vi "ForkOpening.vi"(9 "Presets":T2, 10 "Buttons":bool[](array[boolean])) -> (2 "Opening":T1)   [LabVIEW 2014]
doc: "Set the fork opening according to the button position. Set ForkOffset too"
uses:
  buttons/PresetValues.ctl
  ForkOpening.ctl
  <vilib>/Rock Robotics/Network Tables/SD Write Number.vi
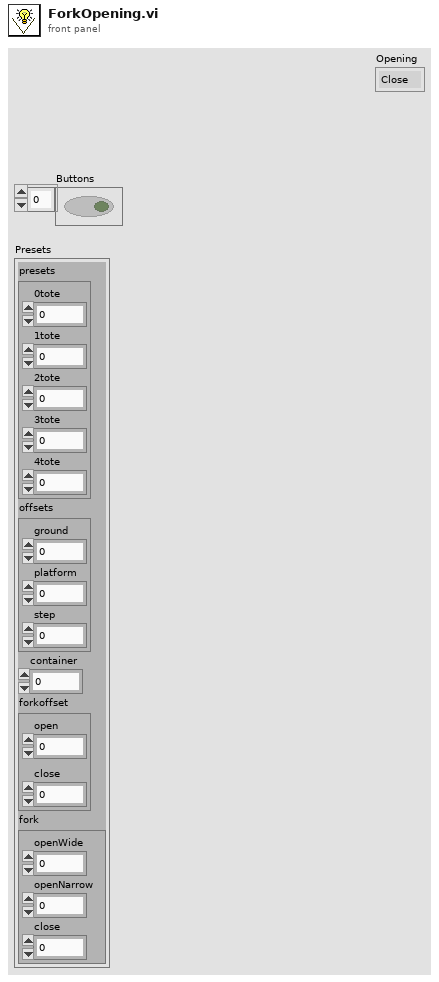
[diagram p1: front panel]
types:
  T1 = typedef "ForkOpening.ctl" = enum16{"Close", "Narrow", "Wide"}
  T2 = typedef "PresetValues.ctl" = cluster{"presets":cluster{"0tote":dbl, "1tote":dbl, "2tote":dbl, "3tote":dbl, "4tote":dbl}, "offsets":cluster{"ground":dbl, "platform":dbl, "step":dbl}, "container":dbl, "forkoffset":cluster{"open":dbl, "close":dbl}, "fork":cluster{"openWide":dbl, "openNarrow":dbl, "close":dbl}}
  T3 = cluster{"openWide":dbl, "openNarrow":dbl, "close":dbl}
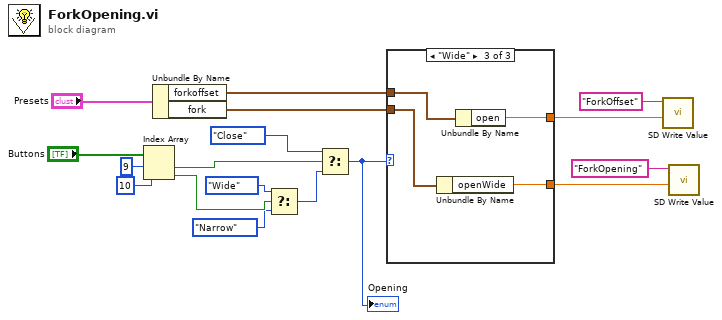
[diagram p0: block diagram]
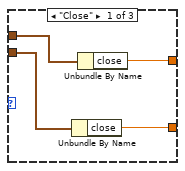
[diagram p2: hidden frame]
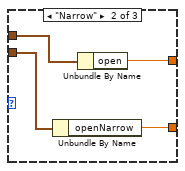
[diagram p3: hidden frame]
diagram:
  n1 = Index Array(array="Buttons", index #1=9 ("index"), index #2=10 ("index")) -> (element #1=w11:bool, element #2=w9:bool)
  n2 = Unbundle By Name("Presets") -> ("forkoffset"=w3:cluster{"open":dbl, "close":dbl}, "fork"=w4:T3)
  n3 = Select(t=ForkOpening."Wide", s=w9, f=ForkOpening."Narrow") -> (s? t:f=w7:T1)
  n4 = Select(t=ForkOpening."Close", s=w11, f=w7) -> (s? t:f=w5:T1)
  "Opening" <- w5
  n5 = case shown="\"Wide\"" w5 {
    tunnel: w4 -> [w21 w25 w29]
    tunnel: w3 -> [w20 w24 w28]
    tunnel: [w19 w23 w27] -> w2
    tunnel: [w18 w22 w26] -> w1
    frame "Close" {
      n6 = Unbundle By Name(w21) -> ("close"=w18:dbl)
      n7 = Unbundle By Name(w20) -> ("close"=w19:dbl)
    }
    frame "Narrow" {
      n8 = Unbundle By Name(w25) -> ("openNarrow"=w22:dbl)
      n9 = Unbundle By Name(w24) -> ("open"=w23:dbl)
    }
    frame "Wide" {
      n10 = Unbundle By Name(w29) -> ("openWide"=w26:dbl)
      n11 = Unbundle By Name(w28) -> ("open"=w27:dbl)
    }
  }
  n12 = call-poly <vilib>:"SD Write Value.vi"("Numeric"=w2, "Name"="ForkOffset") -> ()  [unwired: 8 in, 2 out]
  n13 = call-poly <vilib>:"SD Write Value.vi"("Numeric"=w1, "Name"="ForkOpening") -> ()  [unwired: 8 in, 2 out]
